vi "Read Move Enum_.vi"(8 "error in (no error)":errorcluster, 11 "Multi Column Listbox in":refnum<class "Multi Column Listbox.lvclass">) -> (0 "error out":errorcluster, 2 "Move Enum?":bool, 3 "Multi Column Listbox out":refnum<class "Multi Column Listbox.lvclass">)   [LabVIEW 2013]
uses:
  Multi Column Listbox.lvclass
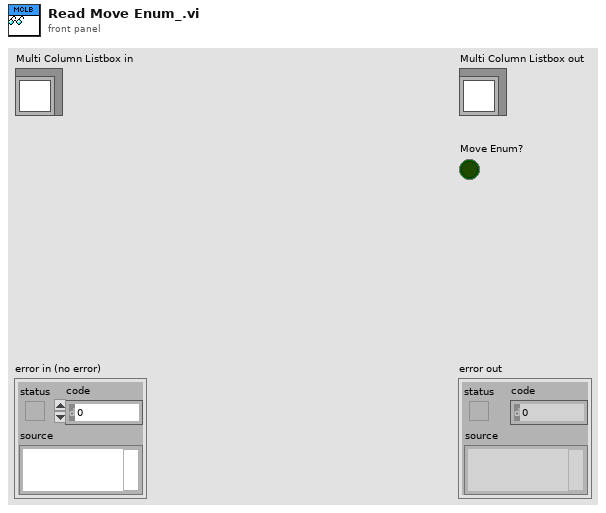
[diagram p1: front panel]
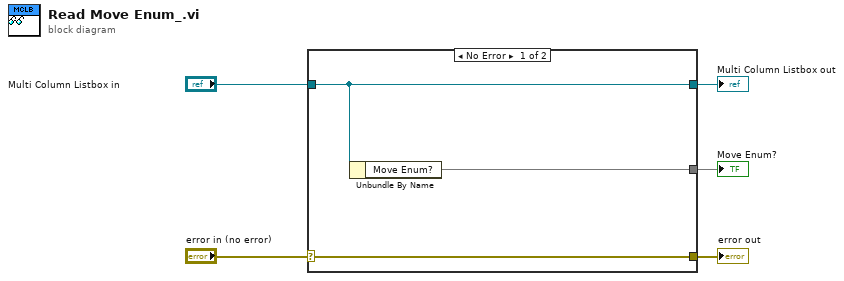
[diagram p0: block diagram]
diagram:
  n1 = case shown="No Error" "error in (no error)" {
    selector: "error in (no error)" -> [w8 w9]
    tunnel: [w8 w9] -> w4
    tunnel: [w7 w10] -> w2
    tunnel: "Multi Column Listbox in" -> [w7 w10]
    tunnel: [w6 _] -> w1
    frame No Error {
      n2 = Unbundle By Name(w7) -> ("Move Enum?"=w6)
    }
    frame Error {
    }
  }
  "error out" <- w4
  "Multi Column Listbox out" <- w2
  "Move Enum?" <- w1
